vi "output.vi"(8 "error in":errorcluster, 10 "data table in":T1, 11 "OPC UA runtime in":refnum<class "OPC UA Server runtime.lvclass">) -> (0 "error out":errorcluster, 2 "data table out":T1, 3 "OPC UA runtime out":refnum<class "OPC UA Server runtime.lvclass">)   [LabVIEW 2013, in "OPC UA Server runtime.lvclass"]
doc: "Provides an interface for writing data to a module at runtime. While this interface performs no operations, a child should provide an override which may write to any open sessions, references, or interfaces."
uses:
  OPC UA Server runtime.lvclass
  <vilib>/NI/Tag Bus/table/data table.ctl
  OPC UA Server runtime.lvclass/OPC UA Server runtime.ctl
  <vilib>/NI/Tag Bus/table/data polymorphs/read one/read Boolean.vi
  <vilib>/NI/Tag Bus/table/data polymorphs/read one/read I8.vi
  <vilib>/NI/Tag Bus/table/data polymorphs/read one/read U8.vi
  <vilib>/NI/Tag Bus/table/data polymorphs/read one/read I16.vi
  <vilib>/NI/Tag Bus/table/data polymorphs/read one/read U16.vi
  <vilib>/NI/Tag Bus/table/data polymorphs/read one/read I32.vi
  <vilib>/NI/Tag Bus/table/data polymorphs/read one/read U32.vi
  <vilib>/NI/Tag Bus/table/data polymorphs/read one/read I64.vi
  <vilib>/NI/Tag Bus/table/data polymorphs/read one/read U64.vi
  <vilib>/NI/Tag Bus/table/data polymorphs/read one/read Single.vi
  <vilib>/NI/Tag Bus/table/data polymorphs/read one/read Double.vi
  <vilib>/NI/Tag Bus/table/data polymorphs/read one/read String.vi
  <vilib>/NI/Tag Bus/table/data polymorphs/read one/read Array of Boolean.vi
  <vilib>/NI/Tag Bus/table/data polymorphs/read one/read Array of I8.vi
  <vilib>/NI/Tag Bus/table/data polymorphs/read one/read Array of U8.vi
  <vilib>/NI/Tag Bus/table/data polymorphs/read one/read Array of I16.vi
  <vilib>/NI/Tag Bus/table/data polymorphs/read one/read Array of U16.vi
  <vilib>/NI/Tag Bus/table/data polymorphs/read one/read Array of I32.vi
  <vilib>/NI/Tag Bus/table/data polymorphs/read one/read Array of U32.vi
  <vilib>/NI/Tag Bus/table/data polymorphs/read one/read Array of I64.vi
  <vilib>/NI/Tag Bus/table/data polymorphs/read one/read Array of U64.vi
  <vilib>/NI/Tag Bus/table/data polymorphs/read one/read Array of Single.vi
  <vilib>/NI/Tag Bus/table/data polymorphs/read one/read Array of Double.vi
  <vilib>/NI/Tag Bus/table/data polymorphs/read one/read Array of String.vi
  <vilib>/OPCUA/server/Write Bool.vi
  <vilib>/OPCUA/server/Write SByte.vi
  <vilib>/OPCUA/server/Write Byte.vi
  <vilib>/OPCUA/server/Write Int16.vi
  <vilib>/OPCUA/server/Write UInt16.vi
  <vilib>/OPCUA/server/Write Int32.vi
  <vilib>/OPCUA/server/Write UInt32.vi
  <vilib>/OPCUA/server/Write Int64.vi
  <vilib>/OPCUA/server/Write UInt64.vi
  <vilib>/OPCUA/server/Write Float.vi
  <vilib>/OPCUA/server/Write Double.vi
  <vilib>/OPCUA/server/Write String.vi
  <vilib>/OPCUA/server/Write Date Time.vi
  <vilib>/OPCUA/server/Write Byte String.vi
  <vilib>/OPCUA/server/Write Bool Array.vi
  <vilib>/OPCUA/server/Write SByte Array.vi
  <vilib>/OPCUA/server/Write Byte Array.vi
  <vilib>/OPCUA/server/Write Int16 Array.vi
  <vilib>/OPCUA/server/Write UInt16 Array.vi
  <vilib>/OPCUA/server/Write Int32 Array.vi
  <vilib>/OPCUA/server/Write UInt32 Array.vi
  <vilib>/OPCUA/server/Write Int64 Array.vi
  <vilib>/OPCUA/server/Write UInt64 Array.vi
  <vilib>/OPCUA/server/Write Float Array.vi
  <vilib>/OPCUA/server/Write Double Array.vi
  <vilib>/OPCUA/server/Write String Array.vi
  <vilib>/OPCUA/server/Write Date Time Array.vi
  <vilib>/OPCUA/server/Write Byte String Array.vi
  <vilib>/Utility/error.llb/Error Cluster From Error Code.vi
  <vilib>/OPCUA/client/Write Bool.vi
  <vilib>/OPCUA/client/Write SByte.vi
  <vilib>/OPCUA/client/Write Byte.vi
  <vilib>/OPCUA/client/Write Int16.vi
  <vilib>/OPCUA/client/Write UInt16.vi
  <vilib>/OPCUA/client/Write Int32.vi
  <vilib>/OPCUA/client/Write UInt32.vi
  <vilib>/OPCUA/client/Write Int64.vi
  <vilib>/OPCUA/client/Write UInt64.vi
  <vilib>/OPCUA/client/Write Float.vi
  <vilib>/OPCUA/client/Write Double.vi
  <vilib>/OPCUA/client/Write String.vi
  <vilib>/OPCUA/client/Write DateTime.vi
  <vilib>/OPCUA/client/Write ByteString.vi
  <vilib>/OPCUA/client/Write Bool Array.vi
  <vilib>/OPCUA/client/Write SByte Array.vi
  <vilib>/OPCUA/client/Write Byte Array.vi
  <vilib>/OPCUA/client/Write Int16 Array.vi
  <vilib>/OPCUA/client/Write UInt16 Array.vi
  <vilib>/OPCUA/client/Write Int32 Array.vi
  <vilib>/OPCUA/client/Write UInt32 Array.vi
  <vilib>/OPCUA/client/Write Int64 Array.vi
  <vilib>/OPCUA/client/Write UInt64 Array.vi
  <vilib>/OPCUA/client/Write Float Array.vi
  <vilib>/OPCUA/client/Write Double Array.vi
  <vilib>/OPCUA/client/Write String Array.vi
  <vilib>/OPCUA/client/Write DateTime Array.vi
  <vilib>/OPCUA/client/Write ByteString Array.vi
  <vilib>/ErrorRing/Error Ring.xnode
  <vilib>/NI/Tag Bus/table/data table.lvlib
  <vilib>/opcua/NI OPC UA Client.lvlib
  <vilib>/opcua/NI OPC UA Server.lvlib
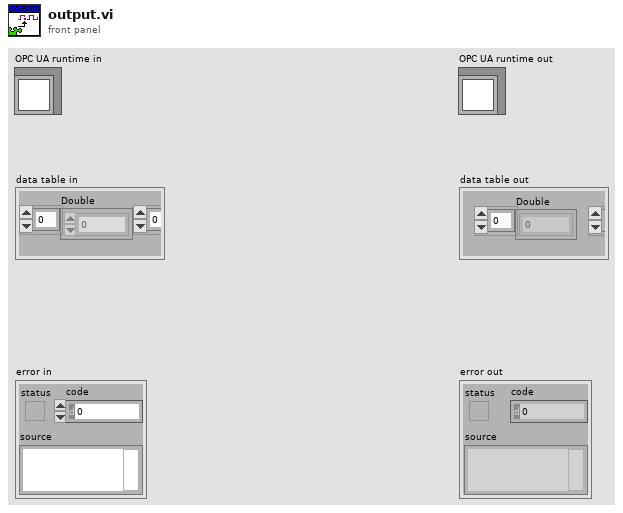
[diagram p1: front panel]
types:
  T1 = typedef "tag bus.lvlib/data table.lvlib/data table.ctl" = cluster{"Double":dbl[], "Single":sgl[], "I64":i64[], "I32":i32[], "I16":i16[], "I8":i8[], "U64":u64[], "U32":u32[], "U16":u16[], "U8":u8[], "Boolean":bool[], "String":string[], "Array of Double":cluster{"DBL Array":dbl[]}[], "Array of Single":cluster{"SGL Array":sgl[]}[], "Array of I64":cluster{"I64 Array":i64[]}[], "Array of I32":cluster{"I32 Array":i32[]}[], "Array of I16":cluster{"I16 Array":i16[]}[], "Array of I8":cluster{"I8 Array":i8[]}[], "Array of U64":cluster{"U64 Array":u64[]}[], "Array of U32":cluster{"U32 Array":u32[]}[], "Array of U16":cluster{"U16 Array":u16[]}[], "Array of U8":cluster{"U8 Array":u8[]}[], "Array of Boolean":cluster{"Boolean Array":bool[]}[], "Array of String":cluster{"String Array":string[]}[]}
  T2 = typedef "tag bus.lvlib/tag descriptor.lvclass/Data Type.ctl" = enum16{"Double", "Single", "I64", "I32", "I16", "I8", "U64", "U32", "U16", "U8", "Boolean", "String", "Array of Double", "Array of Single", "Array of I64", "Array of I32", "Array of I16", "Array of I8", "Array of U64", "Array of U32", "Array of U16", "Array of U8", "Array of Boolean", "Array of String"}
  T3 = typedef "OPC UA Server configuration.lvclass/OPC UA Data Type.ctl" = u16
  T4 = cluster{"DCAF Data Type":T2, "Index":i32, "Node Path":string, "OPC UA Data Type":T3}[]
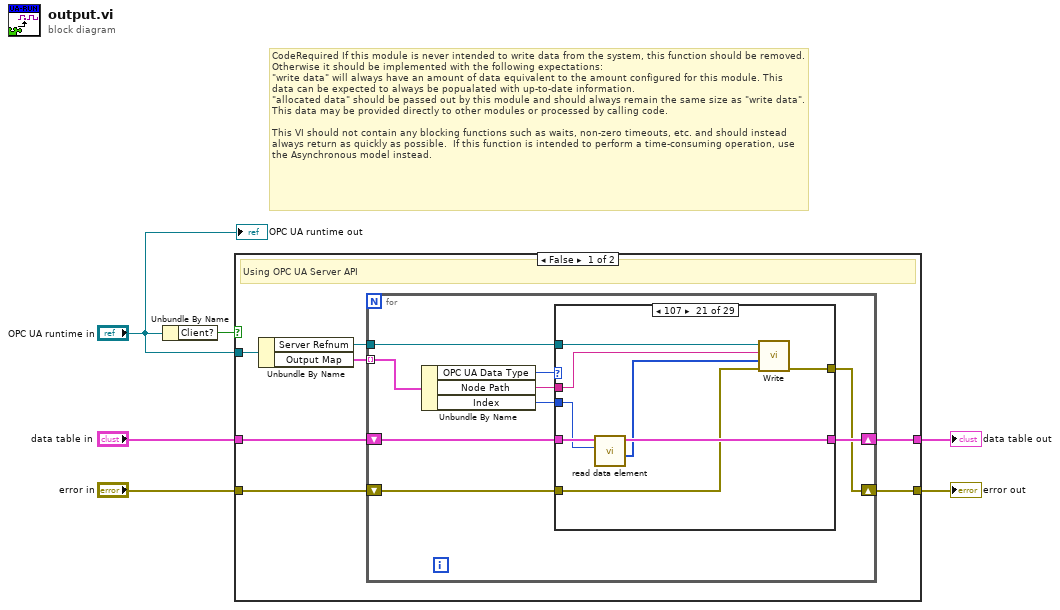
[diagram p0: block diagram]
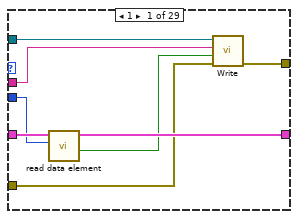
[diagram p2: hidden frame]
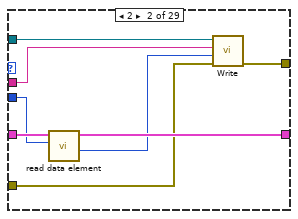
[diagram p3: hidden frame]
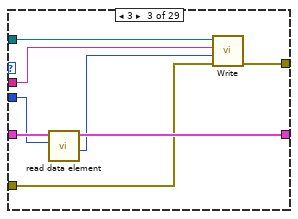
[diagram p4: hidden frame]
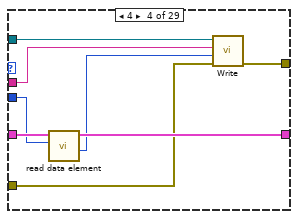
[diagram p5: hidden frame]
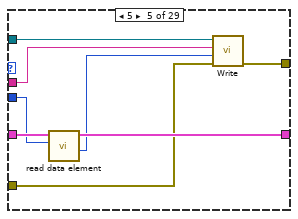
[diagram p6: hidden frame]
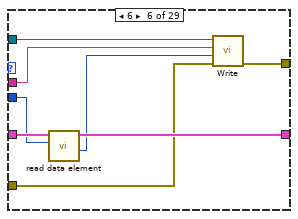
[diagram p7: hidden frame]
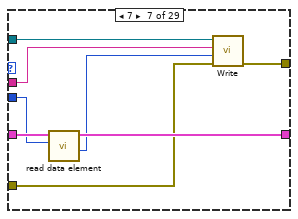
[diagram p8: hidden frame]
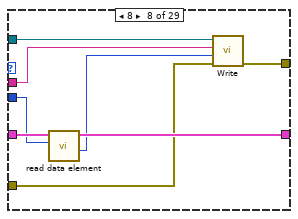
[diagram p9: hidden frame]
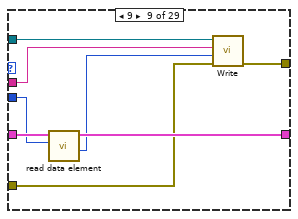
[diagram p10: hidden frame]
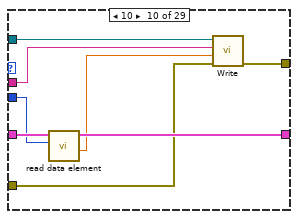
[diagram p11: hidden frame]
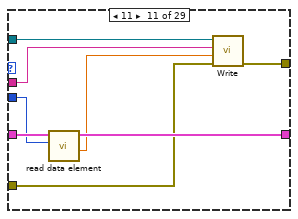
[diagram p12: hidden frame]
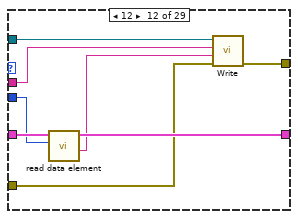
[diagram p13: hidden frame]
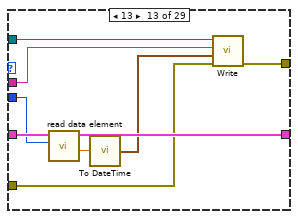
[diagram p14: hidden frame]
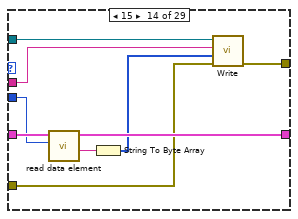
[diagram p15: hidden frame]
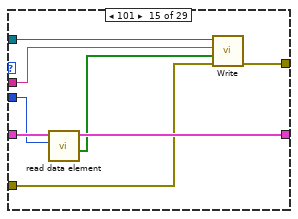
[diagram p16: hidden frame]
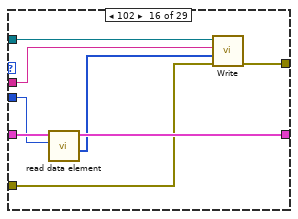
[diagram p17: hidden frame]
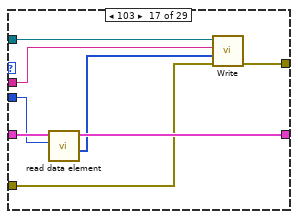
[diagram p18: hidden frame]
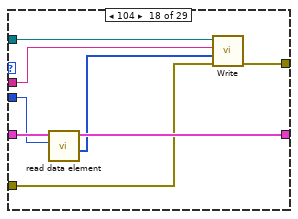
[diagram p19: hidden frame]
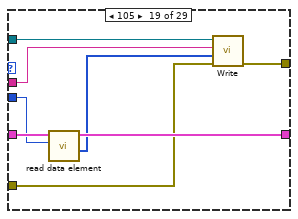
[diagram p20: hidden frame]
diagram:
  # "CodeRequired If this module is never intended to write data from the system, this function should be removed. Otherwise it should be implemented with the following expectations:\n\"write data\" will always have an amount of data equivalent to the amount configured for this module. This data can be expected to always be popualated with up-to-date information.\n\"allocated data\" should be passed out by this module and should always remain the same size as \"write data\". This data may be provided directly to other modules or processed by calling code.\n\nThis VI should not contain any blocking functions such as waits, non-zero timeouts, etc. and should instead always return as quickly as possible.  If this function is intended to perform a time-consuming operation, use the Asynchronous model instead."
  n1 = Unbundle By Name("OPC UA runtime in") -> ("Client?"=w6:bool)
  n2 = case shown="False" w6 {
    tunnel: "OPC UA runtime in" -> [w13 w266]
    tunnel: "data table in" -> [w9 w263]
    tunnel: "error in" -> [w8 w262]
    tunnel: [w10 w261] -> w2
    tunnel: [w7 w260] -> w3
    frame False {
      # "Using OPC UA Server API"
      n3 = Unbundle By Name(w13) -> ("Server Refnum"=w11:refnum<k21>, "Output Map"=w12:T4)
      n4 = for {
        tunnel: w11 -> [w16]
        tunnel: w12 -> [w22] mode=indexing
        shift-right: [w15] -> w7
        shift-left: w8 -> [w18]
        shift-right: [w19] -> w10
        shift-left: w9 -> [w20]
        n5 = Unbundle By Name(w22) -> ("OPC UA Data Type"=w21:T3, "Node Path"=w14:string, "Index"=w17:i32)
        n6 = case shown="107" w21 {
          tunnel: w20 -> [w30 w38 w46 w54 w62 w70 w78 w86 w94 w102 w110 w118 w127 w136 w144 w152 w160 w168 w176 w184 w192 w200 w208 w216 w224 w232 w241 w250 w253]
          tunnel: [w29 w37 w45 w53 w61 w69 w77 w85 w93 w101 w109 w117 w126 w135 w143 w151 w159 w167 w175 w183 w191 w199 w207 w215 w223 w231 w240 w249 w253] -> w19
          tunnel: w18 -> [w25 w33 w41 w49 w57 w65 w73 w81 w89 w97 w105 w113 w122 w131 w139 w147 w155 w163 w171 w179 w187 w195 w203 w211 w219 w227 w236 w245 _]
          tunnel: w17 -> [w28 w36 w44 w52 w60 w68 w76 w84 w92 w100 w108 w116 w125 w134 w142 w150 w158 w166 w174 w182 w190 w198 w206 w214 w222 w230 w239 w248 _]
          tunnel: w16 -> [w27 w35 w43 w51 w59 w67 w75 w83 w91 w99 w107 w115 w124 w133 w141 w149 w157 w165 w173 w181 w189 w197 w205 w213 w221 w229 w238 w247 _]
          tunnel: [w26 w34 w42 w50 w58 w66 w74 w82 w90 w98 w106 w114 w123 w132 w140 w148 w156 w164 w172 w180 w188 w196 w204 w212 w220 w228 w237 w246 w254] -> w15
          tunnel: w14 -> [w24 w32 w40 w48 w56 w64 w72 w80 w88 w96 w104 w112 w121 w130 w138 w146 w154 w162 w170 w178 w186 w194 w202 w210 w218 w226 w235 w244 _]
          frame 1 {
            n7 = call-poly <vilib>:"read data element.vi"("index"=w28, "data table in"=w30) -> ("value"=w23:bool, "data table out"=w29:T1)  [unwired: 8 in]
            n8 = call-poly <vilib>:"Write.vi"("error in (no error)"=w25, "value"=w23, "node path"=w24, "OPC UA server refnum in"=w27) -> ("error out"=w26:errorcluster)  [unwired: 6 in, 1 out]
          }
          frame 2 {
            n9 = call-poly <vilib>:"read data element.vi"("index"=w36, "data table in"=w38) -> ("value"=w31:i8, "data table out"=w37:T1)  [unwired: 8 in]
            n10 = call-poly <vilib>:"Write.vi"("error in (no error)"=w33, "value"=w31, "node path"=w32, "OPC UA server refnum in"=w35) -> ("error out"=w34:errorcluster)  [unwired: 6 in, 1 out]
          }
          frame 3 {
            n11 = call-poly <vilib>:"read data element.vi"("index"=w44, "data table in"=w46) -> ("value"=w39:u8, "data table out"=w45:T1)  [unwired: 8 in]
            n12 = call-poly <vilib>:"Write.vi"("error in (no error)"=w41, "value"=w39, "node path"=w40, "OPC UA server refnum in"=w43) -> ("error out"=w42:errorcluster)  [unwired: 6 in, 1 out]
          }
          frame 4 {
            n13 = call-poly <vilib>:"read data element.vi"("index"=w52, "data table in"=w54) -> ("value"=w47:i16, "data table out"=w53:T1)  [unwired: 8 in]
            n14 = call-poly <vilib>:"Write.vi"("error in (no error)"=w49, "value"=w47, "node path"=w48, "OPC UA server refnum in"=w51) -> ("error out"=w50:errorcluster)  [unwired: 6 in, 1 out]
          }
          frame 5 {
            n15 = call-poly <vilib>:"read data element.vi"("index"=w60, "data table in"=w62) -> ("value"=w55:u16, "data table out"=w61:T1)  [unwired: 8 in]
            n16 = call-poly <vilib>:"Write.vi"("error in (no error)"=w57, "value"=w55, "node path"=w56, "OPC UA server refnum in"=w59) -> ("error out"=w58:errorcluster)  [unwired: 6 in, 1 out]
          }
          frame 6 {
            n17 = call-poly <vilib>:"read data element.vi"("index"=w68, "data table in"=w70) -> ("value"=w63:i32, "data table out"=w69:T1)  [unwired: 8 in]
            n18 = call-poly <vilib>:"Write.vi"("error in (no error)"=w65, "value"=w63, "node path"=w64, "OPC UA server refnum in"=w67) -> ("error out"=w66:errorcluster)  [unwired: 6 in, 1 out]
          }
          frame 7 {
            n19 = call-poly <vilib>:"read data element.vi"("index"=w76, "data table in"=w78) -> ("value"=w71:u32, "data table out"=w77:T1)  [unwired: 8 in]
            n20 = call-poly <vilib>:"Write.vi"("error in (no error)"=w73, "value"=w71, "node path"=w72, "OPC UA server refnum in"=w75) -> ("error out"=w74:errorcluster)  [unwired: 6 in, 1 out]
          }
          frame 8 {
            n21 = call-poly <vilib>:"read data element.vi"("index"=w84, "data table in"=w86) -> ("value"=w79:i64, "data table out"=w85:T1)  [unwired: 8 in]
            n22 = call-poly <vilib>:"Write.vi"("error in (no error)"=w81, "value"=w79, "node path"=w80, "OPC UA server refnum in"=w83) -> ("error out"=w82:errorcluster)  [unwired: 6 in, 1 out]
          }
          frame 9 {
            n23 = call-poly <vilib>:"read data element.vi"("index"=w92, "data table in"=w94) -> ("value"=w87:u64, "data table out"=w93:T1)  [unwired: 8 in]
            n24 = call-poly <vilib>:"Write.vi"("error in (no error)"=w89, "value"=w87, "node path"=w88, "OPC UA server refnum in"=w91) -> ("error out"=w90:errorcluster)  [unwired: 6 in, 1 out]
          }
          frame 10 {
            n25 = call-poly <vilib>:"read data element.vi"("index"=w100, "data table in"=w102) -> ("value"=w95:sgl, "data table out"=w101:T1)  [unwired: 8 in]
            n26 = call-poly <vilib>:"Write.vi"("error in (no error)"=w97, "value"=w95, "node path"=w96, "OPC UA server refnum in"=w99) -> ("error out"=w98:errorcluster)  [unwired: 6 in, 1 out]
          }
          frame 11 {
            n27 = call-poly <vilib>:"read data element.vi"("index"=w108, "data table in"=w110) -> ("value"=w103:dbl, "data table out"=w109:T1)  [unwired: 8 in]
            n28 = call-poly <vilib>:"Write.vi"("error in (no error)"=w105, "value"=w103, "node path"=w104, "OPC UA server refnum in"=w107) -> ("error out"=w106:errorcluster)  [unwired: 6 in, 1 out]
          }
          frame 12 {
            n29 = call-poly <vilib>:"read data element.vi"("index"=w116, "data table in"=w118) -> ("value"=w111:string, "data table out"=w117:T1)  [unwired: 8 in]
            n30 = call-poly <vilib>:"Write.vi"("error in (no error)"=w113, "value"=w111, "node path"=w112, "OPC UA server refnum in"=w115) -> ("error out"=w114:errorcluster)  [unwired: 6 in, 1 out]
          }
          frame 13 {
            n31 = call-poly <vilib>:"read data element.vi"("index"=w125, "data table in"=w127) -> ("value"=w120:dbl, "data table out"=w126:T1)  [unwired: 8 in]
            n32 = call "To DateTime.vi"("Formatted DateTime"=w120) -> ("Time Stamp"=w119:timestamp)
            n33 = call-poly <vilib>:"Write.vi"("error in (no error)"=w122, "value"=w119, "node path"=w121, "OPC UA server refnum in"=w124) -> ("error out"=w123:errorcluster)  [unwired: 6 in, 1 out]
          }
          frame 15 {
            n34 = call-poly <vilib>:"read data element.vi"("index"=w134, "data table in"=w136) -> ("value"=w129:string, "data table out"=w135:T1)  [unwired: 8 in]
            n35 = String To Byte Array(string=w129) -> (unsigned byte array=w128:u8[])
            n36 = call-poly <vilib>:"Write.vi"("error in (no error)"=w131, "value"=w128, "node path"=w130, "OPC UA server refnum in"=w133) -> ("error out"=w132:errorcluster)  [unwired: 6 in, 1 out]
          }
          frame 101 {
            n37 = call-poly <vilib>:"read data element.vi"("index"=w142, "data table in"=w144) -> ("value"=w137:bool[], "data table out"=w143:T1)  [unwired: 8 in]
            n38 = call-poly <vilib>:"Write.vi"("error in (no error)"=w139, "value"=w137, "node path"=w138, "OPC UA server refnum in"=w141) -> ("error out"=w140:errorcluster)  [unwired: 6 in, 1 out]
          }
          frame 102 {
            n39 = call-poly <vilib>:"read data element.vi"("index"=w150, "data table in"=w152) -> ("value"=w145:i8[], "data table out"=w151:T1)  [unwired: 8 in]
            n40 = call-poly <vilib>:"Write.vi"("error in (no error)"=w147, "value"=w145, "node path"=w146, "OPC UA server refnum in"=w149) -> ("error out"=w148:errorcluster)  [unwired: 6 in, 1 out]
          }
          frame 103 {
            n41 = call-poly <vilib>:"read data element.vi"("index"=w158, "data table in"=w160) -> ("value"=w153:u8[], "data table out"=w159:T1)  [unwired: 8 in]
            n42 = call-poly <vilib>:"Write.vi"("error in (no error)"=w155, "value"=w153, "node path"=w154, "OPC UA server refnum in"=w157) -> ("error out"=w156:errorcluster)  [unwired: 6 in, 1 out]
          }
          frame 104 {
            n43 = call-poly <vilib>:"read data element.vi"("index"=w166, "data table in"=w168) -> ("value"=w161:i16[], "data table out"=w167:T1)  [unwired: 8 in]
            n44 = call-poly <vilib>:"Write.vi"("error in (no error)"=w163, "value"=w161, "node path"=w162, "OPC UA server refnum in"=w165) -> ("error out"=w164:errorcluster)  [unwired: 6 in, 1 out]
          }
          frame 105 {
            n45 = call-poly <vilib>:"read data element.vi"("index"=w174, "data table in"=w176) -> ("value"=w169:u16[], "data table out"=w175:T1)  [unwired: 8 in]
            n46 = call-poly <vilib>:"Write.vi"("error in (no error)"=w171, "value"=w169, "node path"=w170, "OPC UA server refnum in"=w173) -> ("error out"=w172:errorcluster)  [unwired: 6 in, 1 out]
          }
          frame 106 {
            n47 = call-poly <vilib>:"read data element.vi"("index"=w182, "data table in"=w184) -> ("value"=w177:i32[], "data table out"=w183:T1)  [unwired: 8 in]
            n48 = call-poly <vilib>:"Write.vi"("error in (no error)"=w179, "value"=w177, "node path"=w178, "OPC UA server refnum in"=w181) -> ("error out"=w180:errorcluster)  [unwired: 6 in, 1 out]
          }
          frame 107 {
            n49 = call-poly <vilib>:"read data element.vi"("index"=w190, "data table in"=w192) -> ("value"=w185:u32[], "data table out"=w191:T1)  [unwired: 8 in]
            n50 = call-poly <vilib>:"Write.vi"("error in (no error)"=w187, "value"=w185, "node path"=w186, "OPC UA server refnum in"=w189) -> ("error out"=w188:errorcluster)  [unwired: 6 in, 1 out]
          }
          frame 108 {
            n51 = call-poly <vilib>:"read data element.vi"("index"=w198, "data table in"=w200) -> ("value"=w193:i64[], "data table out"=w199:T1)  [unwired: 8 in]
            n52 = call-poly <vilib>:"Write.vi"("error in (no error)"=w195, "value"=w193, "node path"=w194, "OPC UA server refnum in"=w197) -> ("error out"=w196:errorcluster)  [unwired: 6 in, 1 out]
          }
          frame 109 {
            n53 = call-poly <vilib>:"read data element.vi"("index"=w206, "data table in"=w208) -> ("value"=w201:u64[], "data table out"=w207:T1)  [unwired: 8 in]
            n54 = call-poly <vilib>:"Write.vi"("error in (no error)"=w203, "value"=w201, "node path"=w202, "OPC UA server refnum in"=w205) -> ("error out"=w204:errorcluster)  [unwired: 6 in, 1 out]
          }
          frame 110 {
            n55 = call-poly <vilib>:"read data element.vi"("index"=w214, "data table in"=w216) -> ("value"=w209:sgl[], "data table out"=w215:T1)  [unwired: 8 in]
            n56 = call-poly <vilib>:"Write.vi"("error in (no error)"=w211, "value"=w209, "node path"=w210, "OPC UA server refnum in"=w213) -> ("error out"=w212:errorcluster)  [unwired: 6 in, 1 out]
          }
          frame 111 {
            n57 = call-poly <vilib>:"read data element.vi"("index"=w222, "data table in"=w224) -> ("value"=w217:dbl[], "data table out"=w223:T1)  [unwired: 8 in]
            n58 = call-poly <vilib>:"Write.vi"("error in (no error)"=w219, "value"=w217, "node path"=w218, "OPC UA server refnum in"=w221) -> ("error out"=w220:errorcluster)  [unwired: 6 in, 1 out]
          }
          frame 112 {
            n59 = call-poly <vilib>:"read data element.vi"("index"=w230, "data table in"=w232) -> ("value"=w225:string[], "data table out"=w231:T1)  [unwired: 8 in]
            n60 = call-poly <vilib>:"Write.vi"("error in (no error)"=w227, "value"=w225, "node path"=w226, "OPC UA server refnum in"=w229) -> ("error out"=w228:errorcluster)  [unwired: 6 in, 1 out]
          }
          frame 113 {
            n61 = call-poly <vilib>:"read data element.vi"("index"=w239, "data table in"=w241) -> ("value"=w234:dbl[], "data table out"=w240:T1)  [unwired: 8 in]
            n62 = call "To DateTime Array.vi"("Formatted DateTime Array"=w234) -> ("DateTime Array"=w233:timestamp[])
            n63 = call-poly <vilib>:"Write.vi"("error in (no error)"=w236, "value"=w233, "node path"=w235, "OPC UA server refnum in"=w238) -> ("error out"=w237:errorcluster)  [unwired: 6 in, 1 out]
          }
          frame 115 {
            n64 = call-poly <vilib>:"read data element.vi"("index"=w248, "data table in"=w250) -> ("value"=w243:string[], "data table out"=w249:T1)  [unwired: 8 in]
            n65 = for {
              tunnel: w243 -> [w252] mode=indexing
              tunnel: [w251] -> w242 mode=indexing
              n66 = String To Byte Array(string=w252) -> (unsigned byte array=w251:u8[])
            }
            n67 = call-poly <vilib>:"Write.vi"("error in (no error)"=w245, "value"=w242, "node path"=w244, "OPC UA server refnum in"=w247) -> ("error out"=w246:errorcluster)  [unwired: 6 in, 1 out]
          }
          frame 0, Default {
            # "invalid data type, throw error"
            n68 = xnode "Error Ring"() -> ("error out"=w254:errorcluster)
          }
        }
      }
    }
    frame True {
      # "Using OPC UA Client API"
      n69 = Unbundle By Name(w266) -> ("Client Refnum"=w265:refnum<k21>, "Output Map"=w264:T4)
      n70 = for {
        tunnel: w265 -> [w271]
        tunnel: w264 -> [w275] mode=indexing
        shift-right: [w268] -> w260
        shift-left: w262 -> [w270]
        shift-right: [w269] -> w261
        shift-left: w263 -> [w273]
        n71 = Unbundle By Name(w275) -> ("OPC UA Data Type"=w274:T3, "Node Path"=w267:string, "Index"=w272:i32)
        n72 = case shown="1" w274 {
          tunnel: w273 -> [w283 w291 w299 w307 w315 w323 w331 w339 w347 w355 w363 w371 w380 w389 w397 w405 w413 w421 w429 w437 w445 w453 w461 w469 w477 w485 w494 w503 w506]
          tunnel: w272 -> [w282 w290 w298 w306 w314 w322 w330 w338 w346 w354 w362 w370 w379 w388 w396 w404 w412 w420 w428 w436 w444 w452 w460 w468 w476 w484 w493 w502 _]
          tunnel: w271 -> [w281 w289 w297 w305 w313 w321 w329 w337 w345 w353 w361 w369 w378 w387 w395 w403 w411 w419 w427 w435 w443 w451 w459 w467 w475 w483 w492 w501 _]
          tunnel: w270 -> [w280 w288 w296 w304 w312 w320 w328 w336 w344 w352 w360 w368 w377 w386 w394 w402 w410 w418 w426 w434 w442 w450 w458 w466 w474 w482 w491 w500 _]
          tunnel: [w279 w287 w295 w303 w311 w319 w327 w335 w343 w351 w359 w367 w376 w385 w393 w401 w409 w417 w425 w433 w441 w449 w457 w465 w473 w481 w490 w499 w506] -> w269
          tunnel: [w278 w286 w294 w302 w310 w318 w326 w334 w342 w350 w358 w366 w375 w384 w392 w400 w408 w416 w424 w432 w440 w448 w456 w464 w472 w480 w489 w498 w507] -> w268
          tunnel: w267 -> [w276 w284 w292 w300 w308 w316 w324 w332 w340 w348 w356 w364 w374 w383 w390 w398 w406 w414 w422 w430 w438 w446 w454 w462 w470 w478 w488 w497 _]
          frame 1 {
            n73 = call-poly <vilib>:"read data element.vi"("index"=w282, "data table in"=w283) -> ("value"=w277:bool, "data table out"=w279:T1)  [unwired: 8 in]
            n74 = call-poly <vilib>:"Write.vi"("error in (no error)"=w280, "value"=w277, "node path"=w276, "OPC UA client refnum in"=w281) -> ("error out"=w278:errorcluster)  [unwired: 5 in, 2 out]
          }
          frame 2 {
            n75 = call-poly <vilib>:"read data element.vi"("index"=w290, "data table in"=w291) -> ("value"=w285:i8, "data table out"=w287:T1)  [unwired: 8 in]
            n76 = call-poly <vilib>:"Write.vi"("error in (no error)"=w288, "value"=w285, "node path"=w284, "OPC UA client refnum in"=w289) -> ("error out"=w286:errorcluster)  [unwired: 5 in, 2 out]
          }
          frame 3 {
            n77 = call-poly <vilib>:"read data element.vi"("index"=w298, "data table in"=w299) -> ("value"=w293:u8, "data table out"=w295:T1)  [unwired: 8 in]
            n78 = call-poly <vilib>:"Write.vi"("error in (no error)"=w296, "value"=w293, "node path"=w292, "OPC UA client refnum in"=w297) -> ("error out"=w294:errorcluster)  [unwired: 5 in, 2 out]
          }
          frame 4 {
            n79 = call-poly <vilib>:"read data element.vi"("index"=w306, "data table in"=w307) -> ("value"=w301:i16, "data table out"=w303:T1)  [unwired: 8 in]
            n80 = call-poly <vilib>:"Write.vi"("error in (no error)"=w304, "value"=w301, "node path"=w300, "OPC UA client refnum in"=w305) -> ("error out"=w302:errorcluster)  [unwired: 5 in, 2 out]
          }
          frame 5 {
            n81 = call-poly <vilib>:"read data element.vi"("index"=w314, "data table in"=w315) -> ("value"=w309:u16, "data table out"=w311:T1)  [unwired: 8 in]
            n82 = call-poly <vilib>:"Write.vi"("error in (no error)"=w312, "value"=w309, "node path"=w308, "OPC UA client refnum in"=w313) -> ("error out"=w310:errorcluster)  [unwired: 5 in, 2 out]
          }
          frame 6 {
            n83 = call-poly <vilib>:"read data element.vi"("index"=w322, "data table in"=w323) -> ("value"=w317:i32, "data table out"=w319:T1)  [unwired: 8 in]
            n84 = call-poly <vilib>:"Write.vi"("error in (no error)"=w320, "value"=w317, "node path"=w316, "OPC UA client refnum in"=w321) -> ("error out"=w318:errorcluster)  [unwired: 5 in, 2 out]
          }
          frame 7 {
            n85 = call-poly <vilib>:"read data element.vi"("index"=w330, "data table in"=w331) -> ("value"=w325:u32, "data table out"=w327:T1)  [unwired: 8 in]
            n86 = call-poly <vilib>:"Write.vi"("error in (no error)"=w328, "value"=w325, "node path"=w324, "OPC UA client refnum in"=w329) -> ("error out"=w326:errorcluster)  [unwired: 5 in, 2 out]
          }
          frame 8 {
            n87 = call-poly <vilib>:"read data element.vi"("index"=w338, "data table in"=w339) -> ("value"=w333:i64, "data table out"=w335:T1)  [unwired: 8 in]
            n88 = call-poly <vilib>:"Write.vi"("error in (no error)"=w336, "value"=w333, "node path"=w332, "OPC UA client refnum in"=w337) -> ("error out"=w334:errorcluster)  [unwired: 5 in, 2 out]
          }
          frame 9 {
            n89 = call-poly <vilib>:"read data element.vi"("index"=w346, "data table in"=w347) -> ("value"=w341:u64, "data table out"=w343:T1)  [unwired: 8 in]
            n90 = call-poly <vilib>:"Write.vi"("error in (no error)"=w344, "value"=w341, "node path"=w340, "OPC UA client refnum in"=w345) -> ("error out"=w342:errorcluster)  [unwired: 5 in, 2 out]
          }
          frame 10 {
            n91 = call-poly <vilib>:"read data element.vi"("index"=w354, "data table in"=w355) -> ("value"=w349:sgl, "data table out"=w351:T1)  [unwired: 8 in]
            n92 = call-poly <vilib>:"Write.vi"("error in (no error)"=w352, "value"=w349, "node path"=w348, "OPC UA client refnum in"=w353) -> ("error out"=w350:errorcluster)  [unwired: 5 in, 2 out]
          }
          frame 11 {
            n93 = call-poly <vilib>:"read data element.vi"("index"=w362, "data table in"=w363) -> ("value"=w357:dbl, "data table out"=w359:T1)  [unwired: 8 in]
            n94 = call-poly <vilib>:"Write.vi"("error in (no error)"=w360, "value"=w357, "node path"=w356, "OPC UA client refnum in"=w361) -> ("error out"=w358:errorcluster)  [unwired: 5 in, 2 out]
          }
          frame 12 {
            n95 = call-poly <vilib>:"read data element.vi"("index"=w370, "data table in"=w371) -> ("value"=w365:string, "data table out"=w367:T1)  [unwired: 8 in]
            n96 = call-poly <vilib>:"Write.vi"("error in (no error)"=w368, "value"=w365, "node path"=w364, "OPC UA client refnum in"=w369) -> ("error out"=w366:errorcluster)  [unwired: 5 in, 2 out]
          }
          frame 13 {
            n97 = call-poly <vilib>:"read data element.vi"("index"=w379, "data table in"=w380) -> ("value"=w373:dbl, "data table out"=w376:T1)  [unwired: 8 in]
            n98 = call "To DateTime.vi"("Formatted DateTime"=w373) -> ("Time Stamp"=w372:timestamp)
            n99 = call-poly <vilib>:"Write.vi"("error in (no error)"=w377, "value"=w372, "node path"=w374, "OPC UA client refnum in"=w378) -> ("error out"=w375:errorcluster)  [unwired: 5 in, 2 out]
          }
          frame 15 {
            n100 = call-poly <vilib>:"read data element.vi"("index"=w388, "data table in"=w389) -> ("value"=w382:string, "data table out"=w385:T1)  [unwired: 8 in]
            n101 = String To Byte Array(string=w382) -> (unsigned byte array=w381:u8[])
            n102 = call-poly <vilib>:"Write.vi"("error in (no error)"=w386, "value"=w381, "node path"=w383, "OPC UA client refnum in"=w387) -> ("error out"=w384:errorcluster)  [unwired: 5 in, 2 out]
          }
          frame 101 {
            n103 = call-poly <vilib>:"read data element.vi"("index"=w396, "data table in"=w397) -> ("value"=w391:bool[], "data table out"=w393:T1)  [unwired: 8 in]
            n104 = call-poly <vilib>:"Write.vi"("error in (no error)"=w394, "value"=w391, "node path"=w390, "OPC UA client refnum in"=w395) -> ("error out"=w392:errorcluster)  [unwired: 5 in, 2 out]
          }
          frame 102 {
            n105 = call-poly <vilib>:"read data element.vi"("index"=w404, "data table in"=w405) -> ("value"=w399:i8[], "data table out"=w401:T1)  [unwired: 8 in]
            n106 = call-poly <vilib>:"Write.vi"("error in (no error)"=w402, "value"=w399, "node path"=w398, "OPC UA client refnum in"=w403) -> ("error out"=w400:errorcluster)  [unwired: 5 in, 2 out]
          }
          frame 103 {
            n107 = call-poly <vilib>:"read data element.vi"("index"=w412, "data table in"=w413) -> ("value"=w407:u8[], "data table out"=w409:T1)  [unwired: 8 in]
            n108 = call-poly <vilib>:"Write.vi"("error in (no error)"=w410, "value"=w407, "node path"=w406, "OPC UA client refnum in"=w411) -> ("error out"=w408:errorcluster)  [unwired: 5 in, 2 out]
          }
          frame 104 {
            n109 = call-poly <vilib>:"read data element.vi"("index"=w420, "data table in"=w421) -> ("value"=w415:i16[], "data table out"=w417:T1)  [unwired: 8 in]
            n110 = call-poly <vilib>:"Write.vi"("error in (no error)"=w418, "value"=w415, "node path"=w414, "OPC UA client refnum in"=w419) -> ("error out"=w416:errorcluster)  [unwired: 5 in, 2 out]
          }
          frame 105 {
            n111 = call-poly <vilib>:"read data element.vi"("index"=w428, "data table in"=w429) -> ("value"=w423:u16[], "data table out"=w425:T1)  [unwired: 8 in]
            n112 = call-poly <vilib>:"Write.vi"("error in (no error)"=w426, "value"=w423, "node path"=w422, "OPC UA client refnum in"=w427) -> ("error out"=w424:errorcluster)  [unwired: 5 in, 2 out]
          }
          frame 106 {
            n113 = call-poly <vilib>:"read data element.vi"("index"=w436, "data table in"=w437) -> ("value"=w431:i32[], "data table out"=w433:T1)  [unwired: 8 in]
            n114 = call-poly <vilib>:"Write.vi"("error in (no error)"=w434, "value"=w431, "node path"=w430, "OPC UA client refnum in"=w435) -> ("error out"=w432:errorcluster)  [unwired: 5 in, 2 out]
          }
          frame 107 {
            n115 = call-poly <vilib>:"read data element.vi"("index"=w444, "data table in"=w445) -> ("value"=w439:u32[], "data table out"=w441:T1)  [unwired: 8 in]
            n116 = call-poly <vilib>:"Write.vi"("error in (no error)"=w442, "value"=w439, "node path"=w438, "OPC UA client refnum in"=w443) -> ("error out"=w440:errorcluster)  [unwired: 5 in, 2 out]
          }
          frame 108 {
            n117 = call-poly <vilib>:"read data element.vi"("index"=w452, "data table in"=w453) -> ("value"=w447:i64[], "data table out"=w449:T1)  [unwired: 8 in]
            n118 = call-poly <vilib>:"Write.vi"("error in (no error)"=w450, "value"=w447, "node path"=w446, "OPC UA client refnum in"=w451) -> ("error out"=w448:errorcluster)  [unwired: 5 in, 2 out]
          }
          frame 109 {
            n119 = call-poly <vilib>:"read data element.vi"("index"=w460, "data table in"=w461) -> ("value"=w455:u64[], "data table out"=w457:T1)  [unwired: 8 in]
            n120 = call-poly <vilib>:"Write.vi"("error in (no error)"=w458, "value"=w455, "node path"=w454, "OPC UA client refnum in"=w459) -> ("error out"=w456:errorcluster)  [unwired: 5 in, 2 out]
          }
          frame 110 {
            n121 = call-poly <vilib>:"read data element.vi"("index"=w468, "data table in"=w469) -> ("value"=w463:sgl[], "data table out"=w465:T1)  [unwired: 8 in]
            n122 = call-poly <vilib>:"Write.vi"("error in (no error)"=w466, "value"=w463, "node path"=w462, "OPC UA client refnum in"=w467) -> ("error out"=w464:errorcluster)  [unwired: 5 in, 2 out]
          }
          frame 111 {
            n123 = call-poly <vilib>:"read data element.vi"("index"=w476, "data table in"=w477) -> ("value"=w471:dbl[], "data table out"=w473:T1)  [unwired: 8 in]
            n124 = call-poly <vilib>:"Write.vi"("error in (no error)"=w474, "value"=w471, "node path"=w470, "OPC UA client refnum in"=w475) -> ("error out"=w472:errorcluster)  [unwired: 5 in, 2 out]
          }
          frame 112 {
            n125 = call-poly <vilib>:"read data element.vi"("index"=w484, "data table in"=w485) -> ("value"=w479:string[], "data table out"=w481:T1)  [unwired: 8 in]
            n126 = call-poly <vilib>:"Write.vi"("error in (no error)"=w482, "value"=w479, "node path"=w478, "OPC UA client refnum in"=w483) -> ("error out"=w480:errorcluster)  [unwired: 5 in, 2 out]
          }
          frame 113 {
            n127 = call-poly <vilib>:"read data element.vi"("index"=w493, "data table in"=w494) -> ("value"=w487:dbl[], "data table out"=w490:T1)  [unwired: 8 in]
            n128 = call "To DateTime Array.vi"("Formatted DateTime Array"=w487) -> ("DateTime Array"=w486:timestamp[])
            n129 = call-poly <vilib>:"Write.vi"("error in (no error)"=w491, "value"=w486, "node path"=w488, "OPC UA client refnum in"=w492) -> ("error out"=w489:errorcluster)  [unwired: 5 in, 2 out]
          }
          frame 115 {
            n130 = call-poly <vilib>:"read data element.vi"("index"=w502, "data table in"=w503) -> ("value"=w496:string[], "data table out"=w499:T1)  [unwired: 8 in]
            n131 = for {
              tunnel: w496 -> [w505] mode=indexing
              tunnel: [w504] -> w495 mode=indexing
              n132 = String To Byte Array(string=w505) -> (unsigned byte array=w504:u8[])
            }
            n133 = call-poly <vilib>:"Write.vi"("error in (no error)"=w500, "value"=w495, "node path"=w497, "OPC UA client refnum in"=w501) -> ("error out"=w498:errorcluster)  [unwired: 5 in, 2 out]
          }
          frame 0, Default {
            # "invalid data type, throw error"
            n134 = xnode "Error Ring"() -> ("error out"=w507:errorcluster)
          }
        }
      }
    }
  }
  "error out" <- w3
  "data table out" <- w2
  "OPC UA runtime out" <- "OPC UA runtime in"
